vi "S8300E_Main_Program_PCBA_MP_WIH.vi"() -> ()   [LabVIEW 2011]
uses:
  Instance           1 33Saved   Konftel_Main_Program_PCBA .vi
  Instance           2 33Saved   Konftel_Main_Program_PCBA .vi
  Instance           7 33Saved   Konftel_Main_Program_PCBA .vi
  Instance           3 33Saved   Konftel_Main_Program_PCBA .vi
  Instance           6 33Saved   Konftel_Main_Program_PCBA .vi
  Instance           5 33Saved   Konftel_Main_Program_PCBA .vi
  Instance           8 33Saved   Konftel_Main_Program_PCBA .vi
panel:
  out "SW Package VER":string
  out "err code 3":i32
  out "error out 3":errorcluster
  out "cancelled 2":bool
  out "shutdown exe file":string
  out "IP POWEROFF EXE FILE":string
  out "uut_logfilename_prefix":string
  out "共花多少分(Spent minutes)":dbl format="%#_6f"
  out "err code 2":i32
  out "error out 2":errorcluster
  out "SFCS Enable ?":bool
  out "err code":i32
  out "error out":errorcluster
  out "cancelled":bool
  out "Target name":string
  out "SN":string
  out "STAGE":string
  out "begin Time":u32
  out "Current Software Version":string
  out "測試程式名稱":string
  out "List run file":string[](array[string])
  in  "Phase  Control":T1(tab)
  out "Totally Test Items":i32
  out "text":string
  out "Test Result Detail":string
  out "ListFile":cluster{"Result":bool, string}[](array[cluster])
  out "測試結果 Result":bool
  # "S8300E Main Program\nS8300E測試主程式"
  # "2015-6-12"
types:
  T1 = enum32{"Script File", "Test Result Detail", "Final Result"}
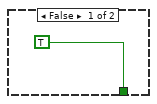
[diagram p5: hidden frame]
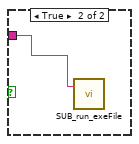
[diagram p7: hidden frame]
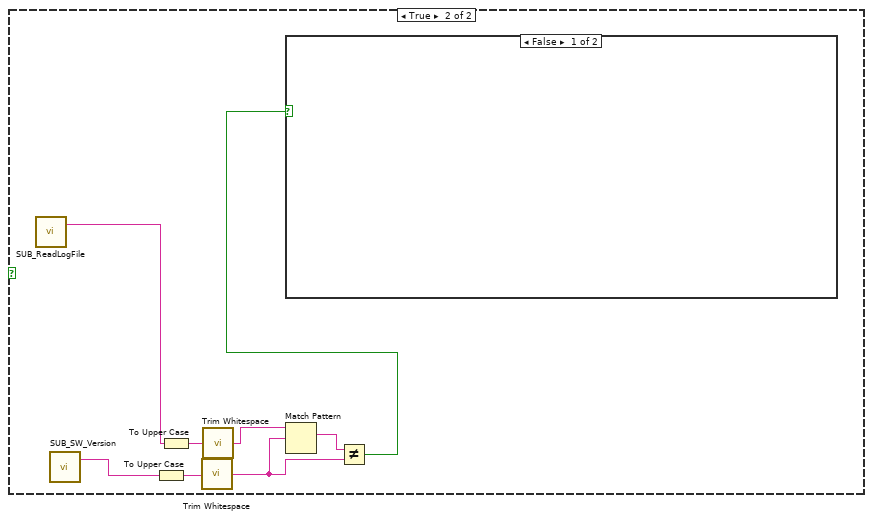
[diagram p9: hidden frame]
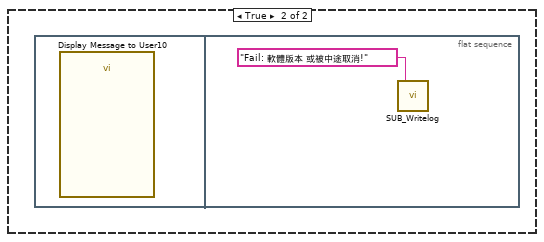
[diagram p10: hidden frame]
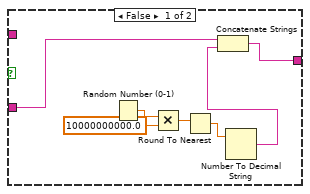
[diagram p12: hidden frame]
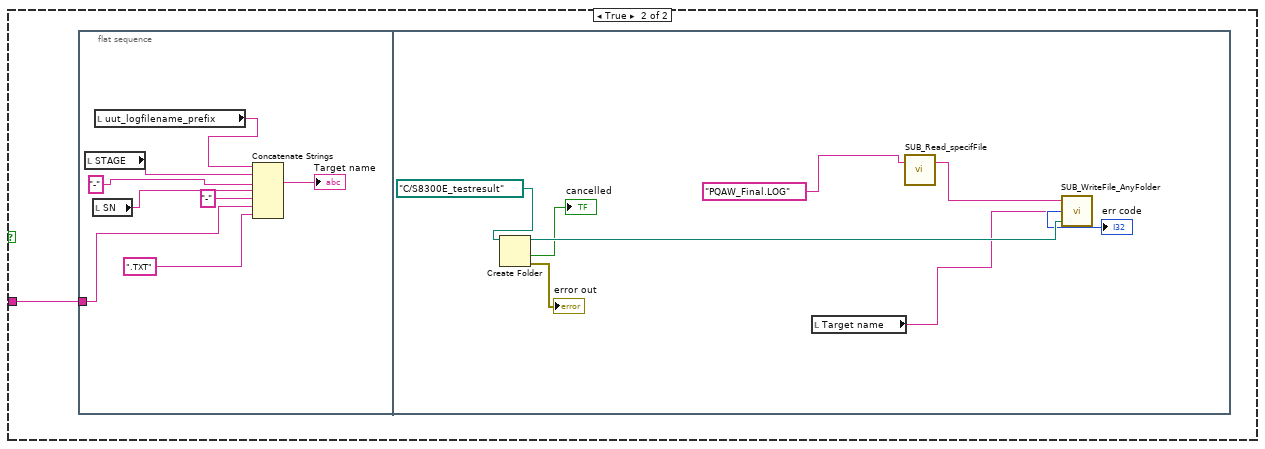
[diagram p13: hidden frame]
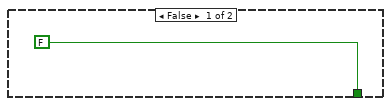
[diagram p15: hidden frame]
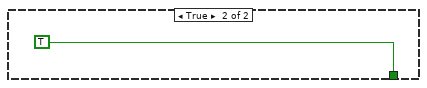
[diagram p16: hidden frame]
diagram:
  n1 = while {
    stop <- FALSE stop-if-true
    n2 = flat-sequence {
      tunnel: [w84] -> w2
      tunnel: w2 -> [w90]
      tunnel: [w90] -> w1
      tunnel: w1 -> [w92]
      tunnel: [w91] -> w7
      tunnel: w7 -> [w216]
      tunnel: [w216] -> w6
      tunnel: w6 -> [w220]
      tunnel: [w220] -> w5
      tunnel: w5 -> [w228]
      tunnel: [w228] -> w4
      tunnel: w4 -> [w229]
      tunnel: [w229] -> w3
      tunnel: w3 -> [w244]
      frame #0 {
        n3 = call "SUB_ReadScript_File.vi"("Script FileName"="S8300E_sfcs_misc.txt") -> ("text"=w12:string, "error out"=w20:errorcluster)  [unwired: 1 in, 1 out]
        n4 = Unbundle By Name(w20) -> ("code"=w22:i32)
        n5 = Equal?(x=w22, y=0) -> ()  [unwired: 1 out]
        n6 = call "SUB_FindSpecificString.vi"("Find this String"="SFCS_SYSTEM_ENABLE=" ("string"), "String data"=w12) -> ("before \"; \" string"=w18:string)  [unwired: 2 in, 1 out]
        n7 = call "SUB_FindSpecificString.vi"("Find this String"="RESULT_LOGFileName_PREFIX=" ("string"), "String data"=w12) -> ("before \"; \" string"=→"uut_logfilename_prefix":string, "Found"=w10:bool)  [unwired: 2 in]
        n8 = call <vilib>:"Trim Whitespace.vi"("string"=w18) -> ("trimmed string"=w19:string)  [unwired: 1 in]
        n9 = call <vilib>:"Trim Whitespace.vi"("string"="YES") -> ("trimmed string"=w17:string)  [unwired: 1 in]
        n10 = To Upper Case(1:w19) -> (0:w15:string)
        n11 = To Upper Case(1:w17) -> (0:w14:string)
        n12 = Equal?(x=w15, y=w14) -> (x = y?=→"SFCS Enable ?":bool)
        n13 = case shown="False" w10 {
          frame False {
            n14 = flat-sequence {
              frame #0 {
                n15 = call "Display Message to User6"() -> ()  [unwired: 10 in, 2 out]
              }
              frame #1 {
                n16 = Stop(stop? (T)=TRUE) -> ()
              }
            }
          }
          frame True {
          }
        }
      }
      frame #1 {
        n17 = Tick Count (ms)() -> (millisecond timer value=→"begin Time":u32)
      }
      frame #2 {
        n18 = property on="共花多少分(Spent minutes)" class="DigNum (strict)"("Visible"=TRUE) -> ()  [unwired: 2 in, 2 out]
      }
      frame #3 {
        n19 = local write "共花多少分(Spent minutes)"(0.0 ("共花多少分(Spent minutes)")) -> ()
      }
      frame #4 {
        n20 = call "SUB_SW_Version.vi"() -> ("Current Software Version"=→"Current Software Version":string)  [unwired: 3 in]
        n21 = local write "測試結果 Result"(FALSE ("Result")) -> ()
        n22 = call "SUB_DELETE_SpecificFile.vi"("Filename to be  Deleted"="SFCS_INFO.LOG" ("name or relative path")) -> ()  [unwired: 2 in, 1 out]
        n23 = call "SUB_DELETE_SpecificFile.vi"("Filename to be  Deleted"="BARCODE.LOG") -> ()  [unwired: 2 in, 1 out]
        n24 = call "SUB_DELETE_SpecificFile.vi"("Filename to be  Deleted"="PQAW_MAC.LOG") -> ()  [unwired: 2 in, 1 out]
        n25 = call "SUB_DELETE_SpecificFile.vi"("Filename to be  Deleted"="SFCS_OperatorID.log") -> ()  [unwired: 2 in, 1 out]
      }
      frame #5 {
        n26 = call "SUB_ReadScript_File.vi"("Script FileName"="S8300E_flow.txt") -> ("text"=→"text":string, "error out"=w42:errorcluster)  [unwired: 1 in, 1 out]
        n27 = local write "Test Result Detail"("") -> ()
        n28 = Unbundle By Name(w42) -> ("code"=w41:i32)
        n29 = local write "Phase  Control"(T1."Test Result Detail" ("Phase  Control")) -> ()
        n30 = Not Equal?(x=w41, y=0) -> (x != y?=w39:bool)
        n31 = case shown="True" w39 {
          frame False {
          }
          frame True {
            n32 = flat-sequence {
              frame #0 {
                n33 = call "Display Message to User"() -> ()  [unwired: 10 in, 2 out]
              }
              frame #1 {
                n34 = local write "Phase  Control"(T1."Final Result" ("Phase  Control")) -> ()
              }
              frame #2 {
                n35 = Stop(stop? (T)=TRUE) -> ()
              }
            }
          }
        }
      }
      frame #6 {
        n36 = call "SUB_Read_specifFile.vi"("name or relative path"="S8300E_sfcs_misc.txt") -> ("text"=w49:string)  [unwired: 1 in, 1 out]
        n37 = call "SUB_FindSpecificString.vi"("Find this String"="IP_POWER_OFF_EXE_FILENAME=", "String data"=w49) -> ("before \"; \" string"=→"IP POWEROFF EXE FILE":string, "Found"=w53:bool)  [unwired: 2 in]
        n38 = call "SUB_FindSpecificString.vi"("Find this String"="S8300E_SW_PACKAGE_VER=", "String data"=w49) -> ("before \"; \" string"=→"SW Package VER":string, "Found"=w46:bool)  [unwired: 2 in]
        n39 = call "SUB_FindSpecificString.vi"("Find this String"="UUT_SHUTDOWN_OFF_EXE_FILENAME=", "String data"=w49) -> ("before \"; \" string"=→"shutdown exe file":string, "Found"=w52:bool)  [unwired: 2 in]
        n40 = And(x=w53, y=w52) -> (x .and. y?=w48:bool)
        n41 = And(x=w48, y=w46) -> (x .and. y?=w47:bool)
        n42 = case shown="False" w47 {
          frame False {
            n43 = flat-sequence {
              frame #0 {
                n44 = call "Display Message to User5"() -> ()  [unwired: 10 in, 2 out]
              }
              frame #1 {
                n45 = Stop(stop? (T)=TRUE) -> ()
              }
            }
          }
          frame True {
          }
        }
      }
      frame #7 {
        n46 = local read "text"() -> (w60:string)
        n47 = while {
          shift-right: [w68] -> _
          shift-left: w60 -> [w77]
          shift-right: [w70] -> _
          shift-left: string[] [] -> [w69]
          stop <- w67 stop-if-true
          n48 = To Upper Case(1:"]" ("string")) -> (0:w64:string)
          n49 = To Upper Case(1:".exe" ("all upper case string")) -> (0:w62:string)
          n50 = To Upper Case(1:w77) -> (0:w66:string)
          n51 = call <vilib>:"Trim Whitespace.vi"("string"=w62) -> ("trimmed string"=w61:string)  [unwired: 1 in]
          n52 = call <vilib>:"Trim Whitespace.vi"("string"=w64) -> ("trimmed string"=w63:string)  [unwired: 1 in]
          n53 = call <vilib>:"Trim Whitespace.vi"("string"=w66) -> ("trimmed string"=w65:string)  [unwired: 1 in]
          n54 = Match Pattern(string=w65, regular expression=w63) -> (after substring=w71:string)  [unwired: 1 in, 3 out]
          n55 = Match Pattern(string=w71, regular expression=w61) -> (match substring=w73:string, after substring=w68:string)  [unwired: 1 in, 2 out]
          n56 = Not Equal?(x=w73, y="") -> (x != y?=w74:bool)
          n57 = case shown="True" w74 {
            tunnel: w71 -> [_ w83]
            tunnel: [_ w80] -> w70
            tunnel: w69 -> [_ w79]
            tunnel: [TRUE _] -> w67
            frame False {
            }
            frame True {
              n58 = Match Pattern(string=w83, regular expression=";") -> (before substring=w81:string)  [unwired: 1 in, 3 out]
              n59 = Build Array (concatenate)(w79, w81) -> (w80:string[])
              "List run file" <- w80
            }
          }
        }
      }
      frame #8 {
        n60 = local read "List run file"() -> (w86:string[])
        n61 = Array Size(array=w86) -> (size(s)=w84:i32)
        n62 = Equal To 0?(x=w84) -> (x = 0?=w85:bool)
        n63 = case shown="True" w85 {
          frame False {
          }
          frame True {
            n64 = flat-sequence {
              frame #0 {
                n65 = call "Display Message to User2"() -> ()  [unwired: 10 in, 2 out]
              }
              frame #1 {
                n66 = local write "Phase  Control"(T1."Final Result" ("Phase  Control")) -> ()
              }
              frame #2 {
                n67 = call "Display Message to User9"() -> ()  [unwired: 10 in, 2 out]
              }
              frame #3 {
                n68 = Stop(stop? (T)=TRUE) -> ()
              }
            }
          }
        }
      }
      frame #9 {
        n69 = call "SUB_DELETE_SpecificFile.vi"("Filename to be  Deleted"="PQAW_Final.LOG") -> ()  [unwired: 2 in, 1 out]
      }
      frame #10 {
        n70 = for {
          N: w92 -> [_]
          shift-right: [w101] -> w91
          shift-left: "" -> [w100]
          i -> [w95]
          n71 = local read "List run file"() -> (w103:string[])
          n72 = Index Array(array=w103, index=w95) -> (element=w102:string)
          n73 = flat-sequence {
            tunnel: w102 -> [w105]
            tunnel: [w105] -> w94
            tunnel: w94 -> [w107]
            tunnel: [w107] -> w96
            tunnel: w96 -> [w110]
            tunnel: w100 -> [w141]
            tunnel: [w142] -> w99
            tunnel: [w142] -> w98
            tunnel: [w142] -> w97
            tunnel: [w153] -> w101
            tunnel: w99 -> [w153]
            tunnel: w98 -> [w149]
            tunnel: w97 -> [w144]
            tunnel: w95 -> [w143]
            frame #0 {
              n74 = Request Deallocation(TRUE ("flag")) -> ()
            }
            frame #1 {
              n75 = call "SUB_DELETE_SpecificFile.vi"("Filename to be  Deleted"="pqaw_err.log" ("Search Filename in Folder")) -> ()  [unwired: 2 in, 1 out]
            }
            frame #2 {
              n76 = call <vilib>:"Trim Whitespace.vi"("string"=w110) -> ("trimmed string"=w108:string)  [unwired: 1 in]
              "測試程式名稱" <- w108
              n77 = call "SUB_SearchFile_inFolder.vi"("Search Filename in Folder"=w108) -> ("File Existing True/Flase"=w109:bool)  [unwired: 1 in]
              n78 = case shown="False" w109 {
                tunnel: w108 -> [w116 w119]
                frame False {
                  n79 = Concatenate Strings("Fail " ("string"), w116, "  ", "File Missing!") -> (w113:string)
                  n80 = flat-sequence {
                    tunnel: w113 -> [w117]
                    tunnel: [w117] -> w112
                    tunnel: w112 -> [w118]
                    frame #0 {
                      n81 = call "Display Message to User3"("Message"=w117) -> ()  [unwired: 9 in, 2 out]
                    }
                    frame #1 {
                      n82 = call "SUB_Writelog.vi"("Pass/Fail"=w118) -> ()  [unwired: 2 in]
                    }
                  }
                }
                frame True {
                  n83 = call "SUB_run_exeFile.vi"("exe filename"=w119) -> ()  [unwired: 2 in, 1 out]
                }
              }
            }
            frame #3 {
              n84 = Request Deallocation(TRUE ("flag")) -> ()
            }
            frame #4 {
              n85 = call "SUB_SearchFile_inFolder.vi"("Search Filename in Folder"="pqaw_err.log") -> ("File Existing True/Flase"=w122:bool)  [unwired: 1 in]
              n86 = case shown="False" w122 {
                frame False {
                  n87 = case shown="True" TRUE {
                    frame False {
                    }
                    frame True {
                      n88 = flat-sequence {
                        frame #0 {
                          n89 = call "Display Message to User11"() -> ()  [unwired: 10 in, 2 out]
                        }
                        frame #1 {
                          n90 = local read "shutdown exe file"() -> (w124:string)
                          n91 = call "SUB_run_exeFile.vi"("exe filename"=w124) -> ()  [unwired: 2 in, 1 out]
                        }
                        frame #2 {
                          n92 = local read "IP POWEROFF EXE FILE"() -> (w125:string)
                          n93 = call "SUB_run_exeFile.vi"("exe filename"=w125) -> ()  [unwired: 2 in, 1 out]
                        }
                        frame #3 {
                          n94 = call "SUB_Writelog.vi"("Pass/Fail"="Fail: Test Program is canceled by Operator !") -> ()  [unwired: 2 in]
                        }
                        frame #4 {
                          n95 = Stop(stop? (T)=TRUE) -> ()
                        }
                      }
                    }
                  }
                }
                frame True {
                  n96 = call "SUB_ReadLogFile.vi"() -> ("text"=w132:string)  [unwired: 2 in, 1 out]
                  n97 = call "SUB_SW_Version.vi"() -> ("Current Software Version"=w131:string)  [unwired: 3 in]
                  n98 = To Upper Case(1:w131) -> (0:w134:string)
                  n99 = To Upper Case(1:w132) -> (0:w135:string)
                  n100 = call <vilib>:"Trim Whitespace.vi"("string"=w134) -> ("trimmed string"=w129:string)  [unwired: 1 in]
                  n101 = call <vilib>:"Trim Whitespace.vi"("string"=w135) -> ("trimmed string"=w133:string)  [unwired: 1 in]
                  n102 = Match Pattern(string=w133, regular expression=w129) -> (match substring=w130:string)  [unwired: 1 in, 3 out]
                  n103 = Not Equal?(x=w130, y=w129) -> (x != y?=w128:bool)
                  n104 = case shown="False" w128 {
                    frame False {
                    }
                    frame True {
                      n105 = flat-sequence {
                        frame #0 {
                          n106 = call "Display Message to User10"() -> ()  [unwired: 10 in, 2 out]
                        }
                        frame #1 {
                          n107 = call "SUB_Writelog.vi"("Pass/Fail"="Fail: 軟體版本 或被中途取消!") -> ()  [unwired: 2 in]
                        }
                      }
                    }
                  }
                }
              }
            }
            frame #5 {
              w138 = "\n"
              n108 = local read "測試程式名稱"() -> (w140:string)
              n109 = call "SUB_ReadLogFile.vi"() -> ("text"=w137:string)  [unwired: 2 in, 1 out]
              n110 = Concatenate Strings(w138, w140, w138) -> (w139:string)
              n111 = Concatenate Strings(w141, w139, w137, w138) -> (w142:string)
              "Test Result Detail" <- w142
            }
            frame #6 {
              n112 = To Upper Case(1:"Fail" ("string")) -> (0:w150:string)
              n113 = To Upper Case(1:w149) -> (0:w152:string)
              n114 = call <vilib>:"Trim Whitespace.vi"("string"=w150) -> ("trimmed string"=w146:string)  [unwired: 1 in]
              n115 = call <vilib>:"Trim Whitespace.vi"("string"=w152) -> ("trimmed string"=w151:string)  [unwired: 1 in]
              n116 = Match Pattern(string=w151, regular expression=w146) -> (match substring=w147:string)  [unwired: 1 in, 3 out]
              n117 = Equal?(x=w147, y=w146) -> (x = y?=w145:bool)
              n118 = case shown="True" w145 {
                tunnel: w144 -> [_ w159]
                tunnel: w143 -> [_ w158]
                frame False {
                }
                frame True {
                  n119 = flat-sequence {
                    tunnel: w159 -> [w161]
                    tunnel: [w161] -> w157
                    tunnel: [w163] -> w156
                    tunnel: w157 -> [w163]
                    tunnel: w156 -> [w184]
                    tunnel: [w184] -> w155
                    tunnel: [w167] -> w154
                    tunnel: w155 -> [w197]
                    tunnel: w154 -> [w195]
                    tunnel: w158 -> [w211]
                    frame #0 {
                      n120 = local read "shutdown exe file"() -> (w160:string)
                      n121 = call "SUB_run_exeFile.vi"("exe filename"=w160) -> ()  [unwired: 2 in, 1 out]
                    }
                    frame #1 {
                      n122 = local read "IP POWEROFF EXE FILE"() -> (w162:string)
                      n123 = call "SUB_run_exeFile.vi"("exe filename"=w162) -> ()  [unwired: 2 in, 1 out]
                    }
                    frame #2 {
                      n124 = call "SUB_Read_specifFile.vi"("name or relative path"="SFCS_INFO.LOG") -> ("error out"=w182:errorcluster, "text"=w181:string)  [unwired: 1 in]
                      n125 = Unbundle By Name(w182) -> ("code"=w179:i32)
                      n126 = local read "uut_logfilename_prefix"() -> (w172:string)
                      n127 = call "SUB_FindSpecificString.vi"("Find this String"="USN=", "String data"=w181) -> ("before \"; \" string"=w171:string, "Found"=w177:bool)  [unwired: 2 in]
                      n128 = call "SUB_GETDateTime_String.vi"() -> ("date/time string"=w164:string)  [unwired: 3 in]
                      n129 = Equal?(x=w179, y=0) -> (x = y?=w174:bool)
                      n130 = Equal?(x=w177, y=TRUE) -> (x = y?=w175:bool)
                      n131 = And(x=w175, y=w174) -> (x .and. y?=w173:bool)
                      n132 = call "SUB_DATETime_Convert.vi"("Input SFCS DateTime String"=w164) -> ("DATE_TIME"=w166:string)
                      n133 = call "SUB_OUT_SpaceString_token.vi"("input string"=w166) -> ("result string"=w165:string)  [unwired: 2 in]
                      n134 = case shown="True" w173 {
                        tunnel: w172 -> [w186 w194]
                        tunnel: w171 -> [_ w193]
                        tunnel: [w185 w192] -> w169
                        frame False {
                          n135 = Random Number (0-1)() -> (number: 0 to 1=w191:dbl)
                          n136 = Multiply(x=w191, y=10000000000.0) -> (x*y=w189:dbl)
                          n137 = Round To Nearest(number=w189) -> (nearest integer value=w188:dbl)
                          n138 = Number To Decimal String(number=w188) -> (decimal integer string=w187:string)  [unwired: 1 in]
                          n139 = Concatenate Strings(w186, w187) -> (w185:string)
                        }
                        frame True {
                          n140 = Concatenate Strings(w194, w193) -> (w192:string)
                        }
                      }
                      n141 = Concatenate Strings(w169, "-" ("string"), w165, "-NG.txt" ("string")) -> (w167:string)
                    }
                    frame #3 {
                      n142 = Create Folder(path (use dialog)=path "C:/S8300E_testresult") -> (created path=w196:path, cancelled=→"cancelled 2":bool, error out=→"error out 3":errorcluster)  [unwired: 2 in]
                      n143 = call "SUB_WriteFinalLog.vi"("Pass/Fail"=w197) -> ()  [unwired: 2 in]
                      n144 = call "SUB_WriteFile_AnyFolder.vi"("base path"=w196, "Filename"=w195, "Text Input"=w197) -> ("err code"=→"err code 3":i32)
                    }
                    frame #4 {
                      n145 = local read "begin Time"() -> (w202:u32)
                      n146 = Tick Count (ms)() -> (millisecond timer value=w208:u32)
                      n147 = Subtract(x=w208, y=w202) -> (x-y=w207:u32)
                      n148 = Divide(x=w207, y=u32 1000) -> (x/y=w205:dbl)
                      n149 = Divide(x=w205, y=60.0) -> (x/y=w203:dbl)
                      n150 = local write "共花多少分(Spent minutes)"(w203) -> ()
                    }
                    frame #5 {
                      n151 = local write "Phase  Control"(T1."Final Result" ("Phase  Control")) -> ()
                    }
                    frame #6 {
                      n152 = local read "Totally Test Items"() -> (w212:i32)
                      n153 = local read "List run file"() -> (w213:string[])
                      n154 = call "SUB_TextRunList_Color.vi"("Current Step"=w211, "Totally Test Items"=w212, "List run file"=w213) -> ("ListFile"=→"ListFile":cluster{"Result":bool, string}[])  [unwired: 2 in]
                    }
                    frame #7 {
                      n155 = call "Display Message to User8"() -> ()  [unwired: 10 in, 2 out]
                    }
                    frame #8 {
                      n156 = Stop(stop? (T)=TRUE) -> ()
                    }
                  }
                }
              }
            }
          }
        }
        "Totally Test Items" <- w92
      }
      frame #11 {
        n157 = property on="測試結果 Result" class="Bool (strict)"("Visible"=FALSE) -> ()  [unwired: 2 in, 2 out]
      }
      frame #12 {
        n158 = local read "List run file"() -> (w218:string[])
        n159 = local read "Totally Test Items"() -> (w219:i32)
        n160 = call "SUB_TextRunList_Color.vi"("Current Step"=w219, "Totally Test Items"=w219, "List run file"=w218) -> ("ListFile"=w217:cluster{"Result":bool, string}[])  [unwired: 2 in]
        n161 = local write "ListFile"(w217) -> ()
      }
      frame #13 {
        n162 = local read "begin Time"() -> (w226:u32)
        n163 = Tick Count (ms)() -> (millisecond timer value=w227:u32)
        n164 = Subtract(x=w227, y=w226) -> (x-y=w225:u32)
        n165 = Divide(x=w225, y=u32 1000) -> (x/y=w223:dbl)
        n166 = Divide(x=w223, y=60.0) -> (x/y=→"共花多少分(Spent minutes)":dbl)
      }
      frame #14 {
        n167 = To Upper Case(1:"fail" ("string")) -> (0:w234:string)
        n168 = To Upper Case(1:w229) -> (0:w236:string)
        n169 = call <vilib>:"Trim Whitespace.vi"("string"=w234) -> ("trimmed string"=w231:string)  [unwired: 1 in]
        n170 = call <vilib>:"Trim Whitespace.vi"("string"=w236) -> ("trimmed string"=w235:string)  [unwired: 1 in]
        n171 = Match Pattern(string=w235, regular expression=w231) -> (match substring=w230:string)  [unwired: 1 in, 3 out]
        n172 = Not Equal?(x=w230, y=w231) -> (x != y?=→"測試結果 Result":bool)
      }
      frame #15 {
        w242 = "\n"
        n173 = local read "共花多少分(Spent minutes)"() -> (w240:dbl)
        n174 = local write "Phase  Control"(T1."Final Result" ("Phase  Control")) -> ()
        n175 = Number To Fractional String(number=w240) -> (F-format string=w239:string)  [unwired: 3 in]
        n176 = Concatenate Strings("Total  Spent Time mins=", w239, "\n") -> (w237:string)
        n177 = Concatenate Strings(w237, w244, w242, "All PASS" ("string"), w242) -> (w245:string)
        n178 = call "SUB_WriteFinalLog.vi"("Pass/Fail"=w245) -> ()  [unwired: 2 in]
      }
      frame #16 {
        n179 = call "SUB_GETDateTime_String.vi"() -> ("date/time string"=w249:string)  [unwired: 3 in]
        n180 = call "SUB_Read_specifFile.vi"("name or relative path"="SFCS_INFO.LOG") -> ("error out"=w262:errorcluster, "text"=w261:string)  [unwired: 1 in]
        n181 = call "SUB_ReadScript_File.vi"("Script FileName"="S8300E_sfcs_misc.txt") -> ("text"=w267:string, "error out"=w268:errorcluster)  [unwired: 1 in, 1 out]
        n182 = Unbundle By Name(w268) -> ("code"=w270:i32)
        n183 = Unbundle By Name(w262) -> ("code"=w259:i32)
        n184 = Equal?(x=w270, y=0) -> (x = y?=w266:bool)
        n185 = call "SUB_DATETime_Convert.vi"("Input SFCS DateTime String"=w249) -> ("DATE_TIME"=w248:string)
        n186 = call "SUB_FindSpecificString.vi"("Find this String"="USN=", "String data"=w261) -> ("before \"; \" string"=→"SN":string, "Found"=w257:bool)  [unwired: 2 in]
        n187 = Equal?(x=w259, y=0) -> (x = y?=w254:bool)
        n188 = call "SUB_FindSpecificString.vi"("Find this String"="SFCS_STAGE=" ("string"), "String data"=w267) -> ("before \"; \" string"=→"STAGE":string, "Found"=w265:bool)  [unwired: 2 in]
        n189 = call "SUB_OUT_SpaceString_token.vi"("input string"=w248) -> ("result string"=w247:string)  [unwired: 2 in]
        n190 = Equal?(x=w257, y=TRUE) -> (x = y?=w255:bool)
        n191 = And(x=w255, y=w254) -> (x .and. y?=w252:bool)
        n192 = And(x=w266, y=w265) -> (x .and. y?=w251:bool)
        n193 = And(x=w251, y=w252) -> (x .and. y?=w250:bool)
        n194 = case shown="False" w250 {
          tunnel: w247 -> [w274 w292]
          frame False {
            n195 = flat-sequence {
              tunnel: [w279] -> w273
              tunnel: w274 -> [w276]
              tunnel: w273 -> [w286]
              frame #0 {
                n196 = Random Number (0-1)() -> (number: 0 to 1=w284:dbl)
                n197 = local read "uut_logfilename_prefix"() -> (w278:string)
                n198 = Multiply(x=w284, y=10000000000.0) -> (x*y=w282:dbl)
                n199 = Round To Nearest(number=w282) -> (nearest integer value=w281:dbl)
                n200 = Number To Decimal String(number=w281) -> (decimal integer string=w280:string)  [unwired: 1 in]
                n201 = Concatenate Strings(w278, w280, "-" ("string"), w276, ".TXT" ("string")) -> (w279:string)
              }
              frame #1 {
                n202 = Create Folder(path (use dialog)=path "C:/S8300E_testresult") -> (created path=w288:path, error out=→"error out 2":errorcluster)  [unwired: 2 in, 1 out]
                n203 = call "SUB_Read_specifFile.vi"("name or relative path"="PQAW_Final.LOG" ("string")) -> ("text"=w289:string)  [unwired: 1 in, 1 out]
                n204 = call "SUB_WriteFile_AnyFolder.vi"("base path"=w288, "Filename"=w286, "Text Input"=w289) -> ("err code"=→"err code 2":i32)
              }
            }
          }
          frame True {
            n205 = flat-sequence {
              tunnel: w292 -> [w294]
              frame #0 {
                n206 = local read "STAGE"() -> (w298:string)
                n207 = local read "SN"() -> (w297:string)
                n208 = local read "uut_logfilename_prefix"() -> (w296:string)
                n209 = Concatenate Strings(w296, w298, "-" ("string"), w297, "-" ("string"), w294, ".TXT" ("string")) -> (→"Target name":string)
              }
              frame #1 {
                n210 = Create Folder(path (use dialog)=path "C:/S8300E_testresult") -> (created path=w308:path, cancelled=→"cancelled":bool, error out=→"error out":errorcluster)  [unwired: 2 in]
                n211 = local read "Target name"() -> (w301:string)
                n212 = call "SUB_Read_specifFile.vi"("name or relative path"="PQAW_Final.LOG" ("string")) -> ("text"=w303:string)  [unwired: 1 in, 1 out]
                n213 = call "SUB_WriteFile_AnyFolder.vi"("base path"=w308, "Filename"=w301, "Text Input"=w303) -> ("err code"=→"err code":i32)
              }
            }
          }
        }
      }
      frame #17 {
        n214 = property on="測試結果 Result" class="Bool (strict)"("Visible"=TRUE) -> ()  [unwired: 2 in, 2 out]
      }
      frame #18 {
        n215 = local read "SFCS Enable ?"() -> (w310:bool)
        n216 = case shown="True" w310 {
          frame False {
          }
          frame True {
            n217 = while {
              stop <- w312 stop-if-true
              n218 = call "SUB_SFCS_SendResult.vi"("ErrorCode"="0", "PASS_Fail (1/0)"=i8 1) -> ("Sent OK ?"=w313:bool)
              n219 = case shown="False" w313 {
                tunnel: [w315 TRUE] -> w312
                frame False {
                  n220 = flat-sequence {
                    tunnel: [w316] -> w315
                    frame #0 {
                      n221 = call "SUB_YESNO.vi"("Debug View"="網路線有插好?", "Status"="上傳系統失敗 或你不上傳 再確認") -> ("yes/no"=w319:enum32{"No Selection", "Yes", "No", "None"})  [unwired: 1 in]
                      n222 = Equal?(x=w319, y=enum32{"No Selection", "Yes", "No", "None"}."No") -> (x = y?=w317:bool)
                      n223 = case shown="True" w317 {
                        tunnel: [FALSE w323] -> w316
                        frame False {
                        }
                        frame True {
                          n224 = flat-sequence {
                            tunnel: [TRUE] -> w323
                            frame #0 {
                              n225 = call "SUB_DELETE_SpecificFile.vi"("Filename to be  Deleted"="PQAW_Final.LOG" ("string")) -> ()  [unwired: 2 in, 1 out]
                            }
                            frame #1 {
                              n226 = call "Display Message to User7"() -> ()  [unwired: 10 in, 2 out]
                            }
                            frame #2 {
                              n227 = Stop(stop? (T)=TRUE) -> ()
                            }
                            frame #3 {
                            }
                          }
                        }
                      }
                    }
                  }
                }
                frame True {
                }
              }
            }
          }
        }
      }
      frame #19 {
        n228 = call "Display Message to User4"() -> ()  [unwired: 10 in, 2 out]
      }
      frame #20 {
        n229 = call "SUB_ASK_YESNO.vi"("Question:"="要繼續測試?選擇Yes繼續.選No 停止測試.") -> ("yes/no"=w330:enum32{"No Selection", "Yes", "No", "None"})  [unwired: 2 in]
        n230 = Equal?(x=w330, y=enum32{"No Selection", "Yes", "No", "None"}."No") -> (x = y?=w328:bool)
        n231 = case shown="True" w328 {
          frame False {
          }
          frame True {
            n232 = Stop(stop? (T)=TRUE) -> ()
          }
        }
      }
    }
  }
